vi "Launch Nested Network Endpoint.vi"(8 "error in":errorcluster, 11 "Study Actor in":refnum<class "Study Actor.lvclass">) -> (0 "error out":errorcluster, 3 "Study Actor out":refnum<class "Study Actor.lvclass">)   [LabVIEW 2023, in "HAL GOOP4.lvlib" / "Study Actor.lvlib" / "Study Actor.lvclass"]
uses:
  Study Actor.lvclass
  <vilib>/ni/Actors/Network Endpoint Actors/Notifying Nested Endpoint/Notifying Nested Endpoint.lvclass
  Study Actor.lvclass/Study Actor.ctl
  <vilib>/ni/Actors/Network Endpoint Actors/Network Endpoint/Network Endpoint/Network Endpoint.lvclass/Network Endpoint.ctl
  <vilib>/ActorFramework/Actor/Actor.lvclass
  <vilib>/ni/Actors/Network Endpoint Actors/Network Endpoint/Network Endpoint/Network Endpoint.lvclass
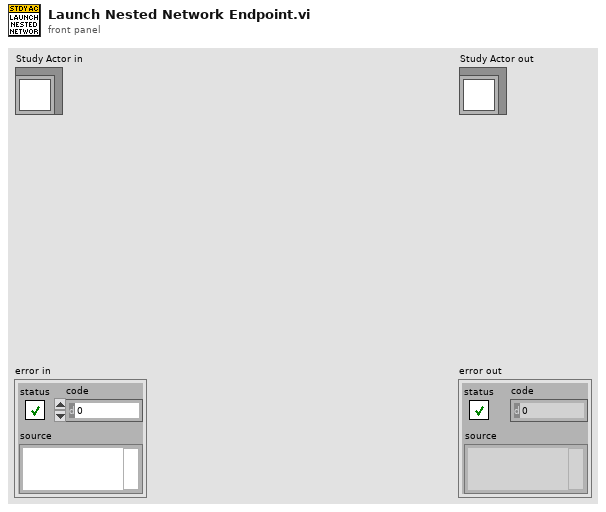
[diagram p1: front panel]
types:
  T1 = map{string, refnum<class "Message Enqueuer.lvclass">}
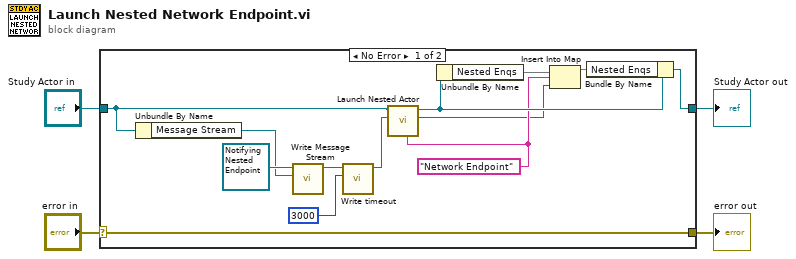
[diagram p0: block diagram]
diagram:
  n1 = case shown="No Error" "error in" {
    selector: "error in" -> [w17 w19]
    tunnel: [w17 w19] -> w3
    tunnel: [w7 w18] -> w1
    tunnel: "Study Actor in" -> [w12 w18]
    frame No Error {
      w6 = "Network Endpoint" ("key")
      n2 = Unbundle By Name(w12) -> ("Message Stream"=w13:refnum<class "Message Stream.lvclass">)
      n3 = call <vilib>:"Write Message Stream.vi"("Message Stream"=w13, "Network Endpoint in"=refnum<class "Notifying Nested Endpoint.lvclass"> refnum ("Notifying Nested Endpoint.lvclass")) -> ("Network Endpoint out"=w15:refnum<class "Notifying Nested Endpoint.lvclass">)  [unwired: 9 in]
      n4 = call <vilib>:"Write timeout.vi"("timeout"=3000, "Network Endpoint in"=w15) -> ("Network Endpoint out"=w11:refnum<class "Notifying Nested Endpoint.lvclass">)  [unwired: 9 in]
      n5 = call <vilib>:"Launch Nested Actor.vi"("Debug Alias"=w6, "Nested Actor"=w11, "Caller Actor in"=w12) -> ("Nested Actor's Enqueuer"=w5:refnum<class "Message Enqueuer.lvclass">, "Caller Actor out"=w8:refnum<class "Study Actor.lvclass">)  [unwired: 6 in, 1 out]
      n6 = Unbundle By Name(w8) -> ("Nested Enqs"=w10:T1)
      n7 = Insert Into Map(map in=w10, key=w6, value=w5) -> (map out=w9:T1)  [unwired: 2 out]
      n8 = Bundle By Name(cluster=w8, "Nested Enqs"=w9) -> (w7:refnum<class "Study Actor.lvclass">)
    }
    frame Error {
    }
  }
  "error out" <- w3
  "Study Actor out" <- w1
